vi "Enable Wash steps.vi"(8 "error in (no error)":errorcluster, 10 "Disabled":T1(ring), 11 "Simulated Entry Console Actor in":refnum<class "Simulated Entry Console Actor.lvclass">) -> (0 "error out":errorcluster, 3 "Simulated Entry Console Actor out":refnum<class "Simulated Entry Console Actor.lvclass">)   [LabVIEW 2019, in "Simulated Entry Console Actor.lvlib" / "Simulated Entry Console Actor.lvclass"]
uses:
  Simulated Entry Console Actor.lvclass
  Simulated Entry Console Actor.lvclass/Simulated Entry Console Actor.ctl
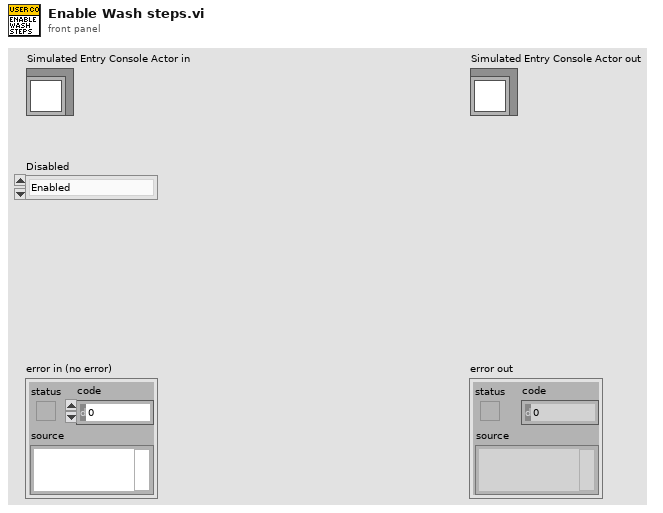
[diagram p1: front panel]
types:
  T1 = enum8{"Enabled", "Disabled", "Disabled and Grayed Out"}
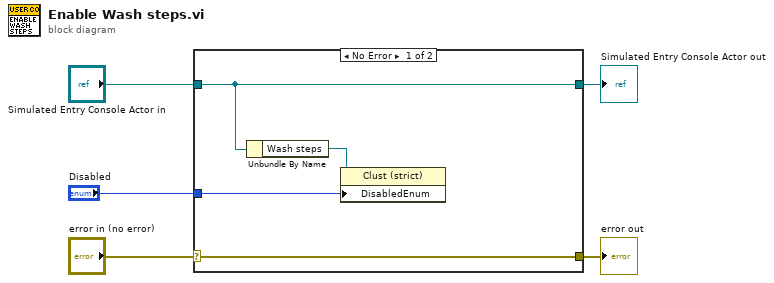
[diagram p0: block diagram]
diagram:
  n1 = case shown="No Error" "error in (no error)" {
    selector: "error in (no error)" -> [w9 w10]
    tunnel: [w9 w10] -> w4
    tunnel: [w8 w11] -> w2
    tunnel: "Simulated Entry Console Actor in" -> [w8 w11]
    tunnel: "Disabled" -> [w6 _]
    frame No Error {
      n2 = Unbundle By Name(w8) -> ("Wash steps"=w7:refnum<vi>)
      n3 = property class="Clust (strict)"(reference=w7, "DisabledEnum"=w6) -> ()  [unwired: 1 in, 2 out]
    }
    frame Error {
    }
  }
  "error out" <- w4
  "Simulated Entry Console Actor out" <- w2
